vi "Root.vi"(11 "BasicTemplater in":refnum<class "BasicTemplater.lvclass">) -> (2 "Templates Root":path, 3 "BasicTemplater out":refnum<class "BasicTemplater.lvclass">)   [LabVIEW 2020, in "HTTP Server.lvlib" / "BasicTemplater.lvclass"]
uses:
  BasicTemplater.lvclass
  BasicTemplater.lvclass/BasicTemplater.ctl
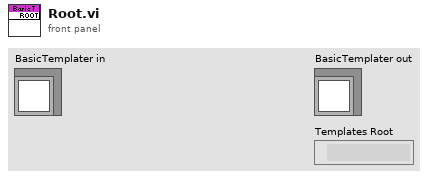
[diagram p1: front panel]
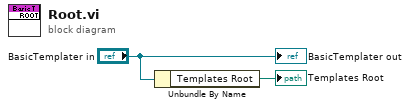
[diagram p0: block diagram]
diagram:
  n1 = Unbundle By Name("BasicTemplater in") -> ("Templates Root"=→"Templates Root":path)
  "BasicTemplater out" <- "BasicTemplater in"
